vi "Set Mouse Lighting.vi"(8 "error in (no error)":errorcluster, 10 "Lighting Zone":T1, 11 "LED Color":u32(colorbox)) -> (0 "error out":errorcluster)   [LabVIEW 2022 SP3, in "Logitech Devices.lvlib"]
uses:
  Logitech Devices.lvlib
  C:/Program Files/LGHUB/sdks/sdk_legacy_led_x86.dll
  TypeDefs/Mouse Lighting Zones.ctl
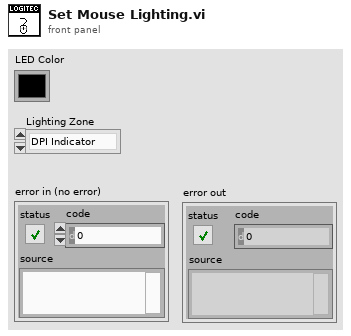
[diagram p1: front panel]
types:
  T1 = typedef "Logitech Devices.lvlib/Mouse Lighting Zones.ctl" = enum8{"DPI Indicator", "Logo"}
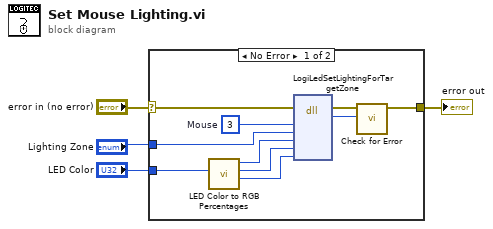
[diagram p0: block diagram]
diagram:
  n1 = case shown="No Error" "error in (no error)" {
    selector: "error in (no error)" -> [w14 w15]
    tunnel: [w7 w15] -> w3
    tunnel: "LED Color" -> [w12 _]
    tunnel: "Lighting Zone" -> [w5 _]
    frame No Error {
      w6 = u8 3  # Mouse
      n2 = call "LED Color to RGB Percentages.vi"("LED Color"=w12) -> ("Blue %"=w9:u8, "Green %"=w10:u8, "Red %"=w11:u8)  [unwired: 8 in]
      n3 = dll-call lib="C:/Program Files/LGHUB/sdks/sdk_legacy_led_x86.dll" fn="LogiLedSetLightingForTargetZone"(error in=w14, "Device Type"=w6, "Zone"=w5, "Red Percentage"=w11, "Green Percentage"=w10, "Blue Percentage"=w9) -> (error out=w8:errorcluster, "return type"=w13:u8)  [unwired: 7 in, 1 out]
      n4 = call "Check for Error.vi"("DLL-call return value"=w13, "error in (no error)"=w8) -> ("error out"=w7:errorcluster)  [unwired: 9 in]
    }
    frame Error {
    }
  }
  "error out" <- w3
